vi "pickDefensiveRobots.vi"(8 "error in (no error)":errorcluster, 11 "Game in":refnum<class "Game.lvclass">) -> (0 "error out":errorcluster, 3 "Game out":refnum<class "Game.lvclass">)   [LabVIEW 2018, in "Game.lvclass"]
uses:
  Game.lvclass
  Game.lvclass/Game.ctl
  Team_class/Team.lvclass/Team.ctl
  Playbook_class/Playbook.lvclass/Playbook.ctl
  TestPlay_class/TestPlay.lvclass/TestPlay.ctl
  Robot_class/roles.ctl
  Role_class/Role.lvclass/Role.ctl
  Robot_class/Robot.lvclass/Robot.ctl
  Robot_class/Write role.vi
  TestPlay_class/Read Roles.vi
  Role_class/Write RobotRef.vi
  TestPlay_class/Write Roles.vi
  Playbook_class/Write defensive_plays.vi
  Playbook_class/Read defensive_plays.vi
  TestPlay_class/Read NumberOfRobots.vi
  Read AllyRef.vi
  Read Referee.vi
  Read Playbook.vi
  Read DefensiveTeam.vi
  Read OffensiveTeam.vi
  Read KeeperTeam.vi
  Team_class/Read KeeperPlay.vi
  Team_class/Read RobotRef.vi
  Team_class/Write RobotRef.vi
  Write DefensiveTeam.vi
  Write Playbook.vi
  Ally_class/Ally.lvclass
  C:/Users/nicolas.oliveira/roboime/SSL_AI/Team_class/Team.lvclass
  TestRole_class/TestRole.lvclass
  C:/Users/nicolas.oliveira/roboime/SSL_AI/Role_class/Role.lvclass
  Referee_class/Referee.lvclass
  Playbook_class/Playbook.lvclass
  Robot_class/Robot.lvclass
  Play_class/Play.lvclass
  TestPlay_class/TestPlay.lvclass
  Role_class/Role.lvclass
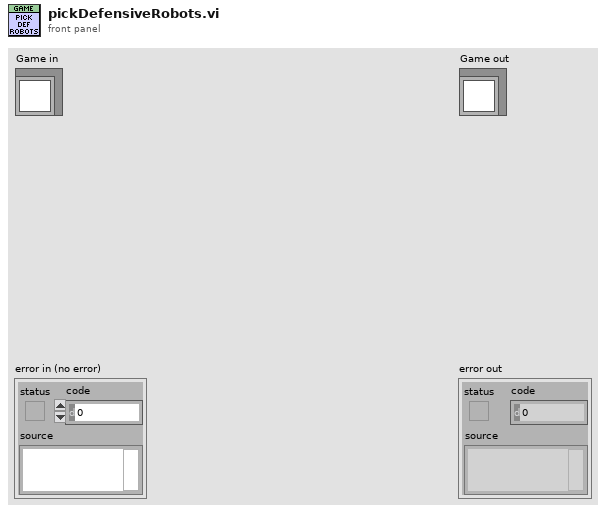
[diagram p1: front panel]
types:
  T1 = typedef "roles.ctl" = enum16{"Halt", "Role", "TestRole"}
  T2 = typedef "KeeperPlay.ctl" = enum16{"NormalGame", "Halt", "Timeout", "PenaltyEnemy", "TestPlay"}
  T3 = cluster{"Play":refnum<class "Play.lvclass">, "TestPlay":refnum<class "TestPlay.lvclass">}
  T4 = cluster{"TestRole 1":refnum<class "TestRole.lvclass">, "Role":refnum<class "Role.lvclass">, "TestRole 2":refnum<class "TestRole.lvclass">, "TestRole 3":refnum<class "TestRole.lvclass">}
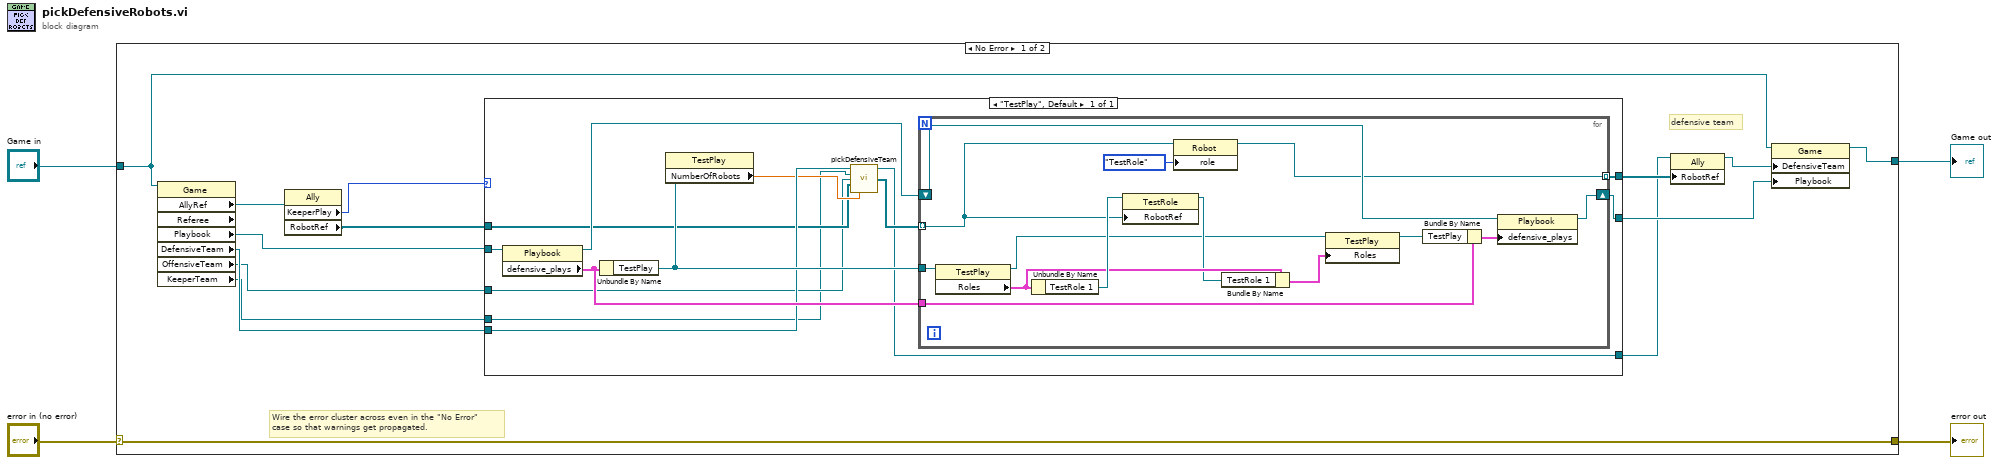
[diagram p0: block diagram]
diagram:
  n1 = case shown="No Error" "error in (no error)" {
    selector: "error in (no error)" -> [w11 w47]
    tunnel: [w11 w47] -> w3
    tunnel: [w12 w46] -> w1
    tunnel: "Game in" -> [w14 w46]
    frame No Error {
      # "defensive team"
      # "Wire the error cluster across even in the \"No Error\"\ncase so that warnings get propagated."
      n2 = property class="Game" props=["AllyRef", "Referee", "Playbook", "DefensiveTeam", "OffensiveTeam", "KeeperTeam"](reference=w14) -> ("AllyRef"=w18:refnum<class "Ally.lvclass">, "Playbook"=w16:refnum<class "Playbook.lvclass">, "DefensiveTeam"=w9:refnum<class "Ally.lvclass">, "OffensiveTeam"=w6:refnum<class "Ally.lvclass">, "KeeperTeam"=w5:refnum<class "Ally.lvclass">)  [unwired: 1 in, 3 out]
      n3 = property class="Ally"(reference=w18) -> ("KeeperPlay"=w17:T2, "RobotRef"=w15:refnum<class "Robot.lvclass">[])  [unwired: 1 in, 2 out]
      n4 = case shown="\"TestPlay\", Default" w17 {
        tunnel: w16 -> [w31]
        tunnel: w15 -> [w23]
        tunnel: [w29] -> w13
        tunnel: [w28] -> w8
        tunnel: w9 -> [w25]
        tunnel: [w21] -> w7
        tunnel: w6 -> [w20]
        tunnel: w5 -> [w19]
        frame "TestPlay", Default {
          n5 = property class="Playbook"(reference=w31) -> (reference out=w26:refnum<class "Playbook.lvclass">, "defensive_plays"=w30:T3)  [unwired: 1 in, 1 out]
          n6 = Unbundle By Name(w30) -> ("TestPlay"=w27:refnum<class "TestPlay.lvclass">)
          n7 = property class="TestPlay"(reference=w27) -> ("NumberOfRobots"=w24:dbl)  [unwired: 1 in, 2 out]
          n8 = call-dynamic "pickDefensiveTeam.vi"("Ally in"=w25, "KeeperTeam"=w19, "OffensiveTeam"=w20, "RobotRef in"=w23, "number_of_robots"=w24) -> ("Ally out"=w21:refnum<class "Ally.lvclass">, "RobotRef"=w22:refnum<class "Robot.lvclass">[])  [unwired: 8 in, 1 out]
          n9 = for {
            tunnel: w30 -> [w40]
            tunnel: [w33] -> w28 mode=indexing
            tunnel: w27 -> [w34]
            tunnel: w22 -> [w32] mode=indexing
            shift-right: [w36] -> w29
            shift-left: w26 -> [w37]
            n10 = property class="TestPlay"(reference=w34) -> (reference out=w41:refnum<class "TestPlay.lvclass">, "Roles"=w44:T4)  [unwired: 1 in, 1 out]
            n11 = Unbundle By Name(w44) -> ("TestRole 1"=w45:refnum<class "TestRole.lvclass">)
            n12 = property class="TestRole"(reference=w45, "RobotRef"=w32) -> (reference out=w43:refnum<class "TestRole.lvclass">)  [unwired: 1 in, 1 out]
            n13 = property class="Robot"(reference=w32, "role"=roles."TestRole") -> (reference out=w33:refnum<class "Robot.lvclass">)  [unwired: 1 in, 1 out]
            n14 = Bundle By Name(cluster=w44, "TestRole 1"=w43) -> (w42:T4)
            n15 = property class="TestPlay"(reference=w41, "Roles"=w42) -> (reference out=w39:refnum<class "TestPlay.lvclass">)  [unwired: 1 in, 1 out]
            n16 = Bundle By Name(cluster=w40, "TestPlay"=w39) -> (w38:T3)
            n17 = property class="Playbook"(reference=w37, "defensive_plays"=w38) -> (reference out=w36:refnum<class "Playbook.lvclass">)  [unwired: 1 in, 1 out]
          }
        }
      }
      n18 = property class="Ally"(reference=w7, "RobotRef"=w8) -> (reference out=w10:refnum<class "Ally.lvclass">)  [unwired: 1 in, 1 out]
      n19 = property class="Game"(reference=w14, "DefensiveTeam"=w10, "Playbook"=w13) -> (reference out=w12:refnum<class "Game.lvclass">)  [unwired: 1 in, 1 out]
    }
    frame Error {
    }
  }
  "error out" <- w3
  "Game out" <- w1
